vi "Toggle.vi"(1 "Boolean":bool) -> (0 "Boolean Out":bool)   [LabVIEW 2018]
doc: "This VI holds a value for the output until the value of the Boolean is switched from true to false. When it is switched it switches the output to the opposite of what it was. In a real life scenario, the value of the output would switch every time the button is pressed."
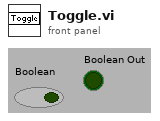
[diagram p1: front panel]
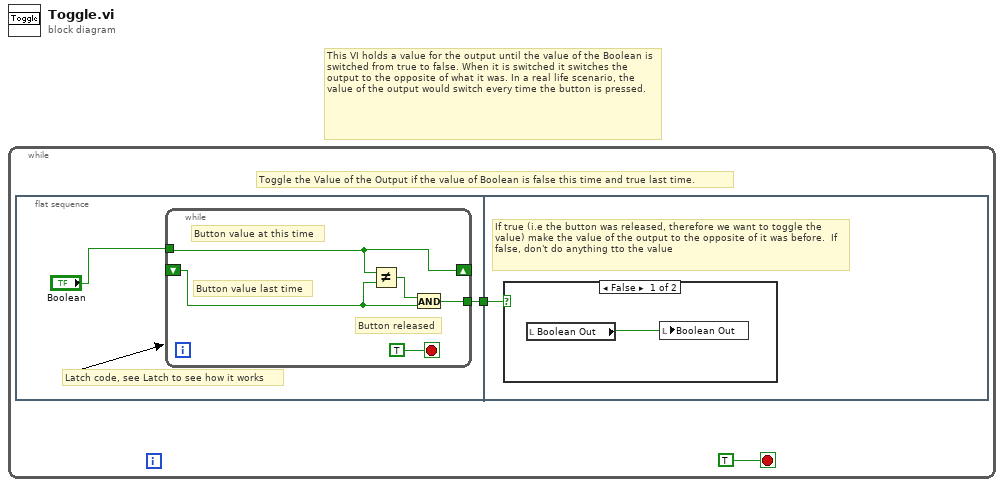
[diagram p0: block diagram]
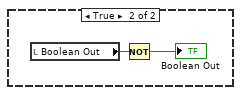
[diagram p2: hidden frame]
diagram:
  # "This VI holds a value for the output until the value of the Boolean is switched from true to false. When it is switched it switches the output to the opposite of what it was. In a real life scenario, the value of the output would switch every time the button is pressed."
  n1 = while {
    stop <- TRUE stop-if-true
    # "Toggle the Value of the Output if the value of Boolean is false this time and true last time."
    n2 = flat-sequence {
      tunnel: [w3] -> w1
      tunnel: w1 -> [w10]
      frame #0 {
        # "Latch code, see Latch to see how it works"
        n3 = while {
          tunnel: [w8] -> w3
          tunnel: "Boolean" -> [w7]
          shift-right: [w7] -> _
          shift-left: _ -> [w6]
          stop <- TRUE ("stop") stop-if-true
          # "Button released"
          # "Button value last time"
          # "Button value at this time"
          n4 = Not Equal?(x=w7, y=w6) -> (x != y?=w9:bool)
          n5 = And(x=w9, y=w6) -> (x .and. y?=w8:bool)
        }
      }
      frame #1 {
        # "If true (i.e the button was released, therefore we want to toggle the value) make the value of the output to the opposite of it was before.  If false, don't do anything tto the value"
        n6 = case shown="False" w10 {
          frame False {
            n7 = local read "Boolean Out"() -> (w11:bool)
            n8 = local write "Boolean Out"(w11) -> ()
          }
          frame True {
            n9 = local read "Boolean Out"() -> (w13:bool)
            n10 = Not(x=w13) -> (.not. x?=→"Boolean Out":bool)
          }
        }
      }
    }
  }
